vi "LoadProfiletest.vi"() -> ()   [LabVIEW 2020]
uses:
  <vilib>/Utility/file.llb/Read Delimited Spreadsheet (DBL).vi
panel:
  out "NHR error out":errorcluster
  out "VISA resource name out":refnum<visa-resource-name>
  in  "Battery Type":enum16{"30Q", "40T"}(ring)
  in  "PS VISA in":refnum<visa-resource-name>
  in  "PS type":enum16{"NHR", "ITECH"}(ring)
  in  "CyclePath":path=path "C:/Users/ga11/Desktop/VI/results/3PtestCharge.lvm" caption="Filename"
  in  "Test Time (s)":dbl format="%#.6g"
  out "Current Step":u32
  out "Time  Elapsed":dbl
  out "Time Step":dbl
  out "Load Output (A)":dbl
  out "Time Ref":dbl
  out "first row 2":dbl[](array[numeric])
  out "first row":dbl[](array[numeric])
  in  "Time file path (seconds)":path
  in  "Load file path (Amps)":path
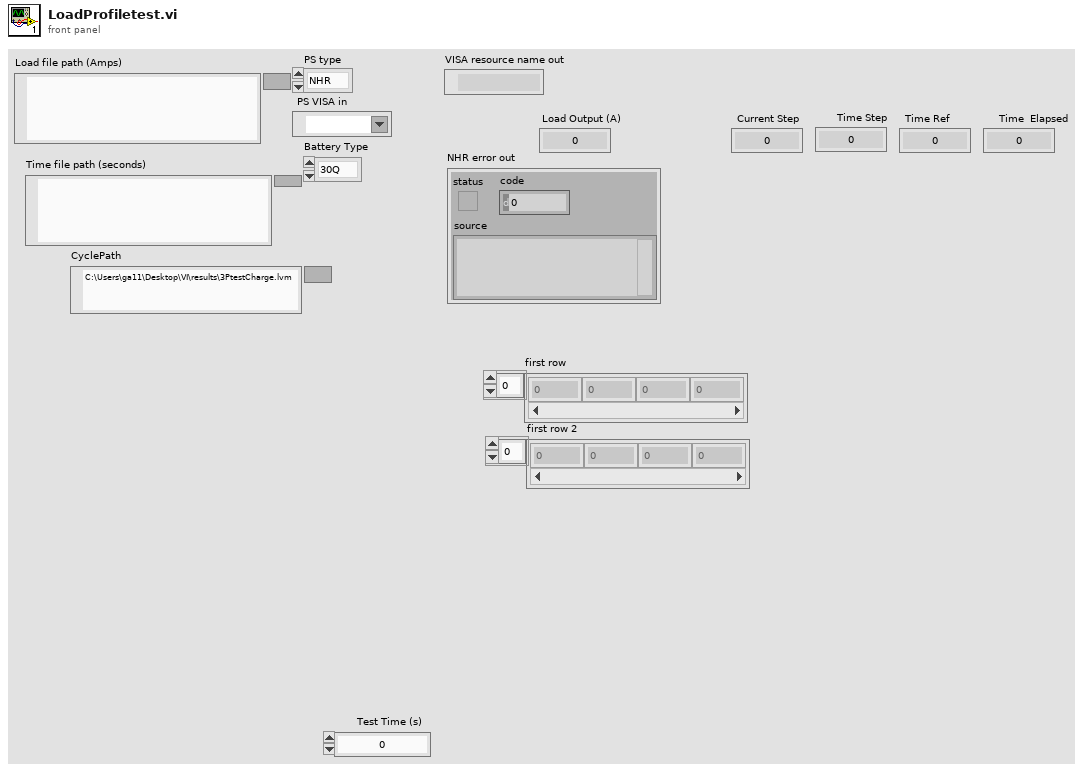
[diagram p1: front panel]
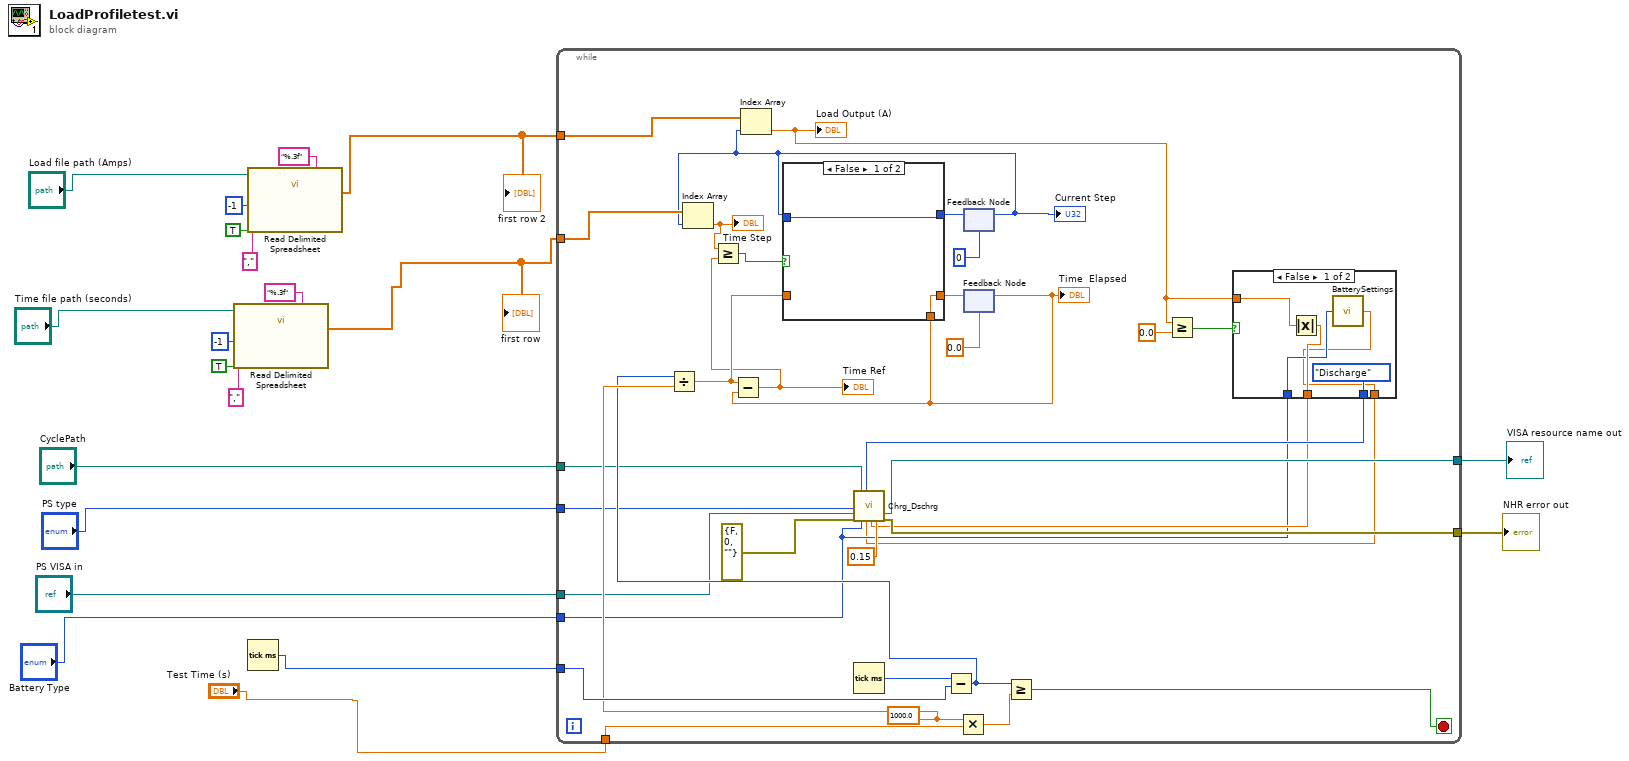
[diagram p0: block diagram]
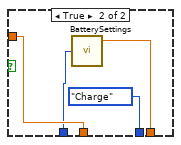
[diagram p2: hidden frame]
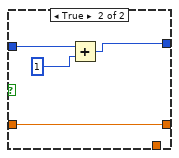
[diagram p3: hidden frame]
diagram:
  n1 = call-poly <vilib>:"Read Delimited Spreadsheet.vi"("file path (dialog if empty)"="Time file path (seconds)", "format (%.3f)"="%.3f", "number of rows (all:-1)"=-1, "transpose? (F)"=TRUE, "delimiter (\\t)"="," ("delimiter (\\t)")) -> ("first row"=w10:dbl[])  [unwired: 5 in, 5 out]
  "first row" <- w10
  n2 = call-poly <vilib>:"Read Delimited Spreadsheet.vi"("file path (dialog if empty)"="Load file path (Amps)", "format (%.3f)"="%.3f", "number of rows (all:-1)"=-1, "transpose? (F)"=TRUE, "delimiter (\\t)"="," ("delimiter (\\t)")) -> ("first row"=w9:dbl[])  [unwired: 5 in, 5 out]
  "first row 2" <- w9
  n3 = Tick Count (ms)() -> (millisecond timer value=w8:u32)
  n4 = while {
    tunnel: w10 -> [w47]
    tunnel: w9 -> [w46]
    tunnel: w8 -> [w43]
    tunnel: "Test Time (s)" -> [w41]
    tunnel: "CyclePath" -> [w33]
    tunnel: "PS type" -> [w32]
    tunnel: "PS VISA in" -> [w31]
    tunnel: "Battery Type" -> [w22]
    tunnel: [w29] -> w2
    tunnel: [w28] -> w1
    stop <- w39 stop-if-true
    w42 = 1000.0
    n5 = Tick Count (ms)() -> (millisecond timer value=w45:u32)
    n6 = Subtract(x=w45, y=w43) -> (x-y=w40:u32)
    n7 = Divide(x=w40, y=w42) -> (x/y=w53:dbl)
    n8 = Multiply(x=w42, y=w41) -> (x*y=w44:dbl)
    n9 = feedback #1(0) -> (w38:i32)
    "Current Step" <- w38
    n10 = Index Array(array=w47, index=w38) -> (element=w35:dbl)
    "Time Step" <- w35
    n11 = Index Array(array=w46, index=w38) -> (element=w24:dbl)
    "Load Output (A)" <- w24
    n12 = feedback #2(0.0) -> (w48:dbl)
    "Time  Elapsed" <- w48
    n13 = Subtract(x=w53, y=w48) -> (x-y=w37:dbl)
    "Time Ref" <- w37
    n14 = Greater Or Equal?(x=w35, y=w37) -> (x >= y?=w36:bool)
    n15 = case shown="False" w36 {
      tunnel: w53 -> [_ w68]
      tunnel: [w64 w68] -> w52
      tunnel: w48 -> [w64 _]
      tunnel: [w63 w66] -> w51
      tunnel: w38 -> [w63 w65]
      frame False {
      }
      frame True {
        n16 = Add(x=w65, y=1) -> (x+y=w66:i32)
      }
    }
    n17 = feedback-in #1(w51) -> ()
    n18 = feedback-in #2(w52) -> ()
    n19 = Greater Or Equal?(x=w40, y=w44) -> (x >= y?=w39:bool)
    n20 = Greater Or Equal?(x=w24, y=0.0) -> (x >= y?=w26:bool)
    n21 = case shown="False" w26 {
      tunnel: [enum8{"Charge", "Discharge"}."Discharge" ("Charge/discharge") enum8{"Charge", "Discharge"}."Charge" ("Charge/discharge")] -> w25
      tunnel: w24 -> [w57 w61]
      tunnel: [w56 w61] -> w23
      tunnel: w22 -> [w55 w60]
      tunnel: [w54 w59] -> w21
      frame False {
        n22 = Absolute Value(x=w57) -> (abs(x)=w56:dbl)
        n23 = call "BatterySettings.vi"("Battery Type"=w55) -> ("Min Voltage (V)"=w54:dbl)  [unwired: 2 in, 2 out]
      }
      frame True {
        n24 = call "BatterySettings.vi"("Battery Type"=w60) -> ("Max Voltage (V)"=w59:dbl)  [unwired: 2 in, 2 out]
      }
    }
    n25 = call "Chrg_Dschrg.vi"("PS type"=w32, "PS VISA in"=w31, "PS error in"=errorcluster {"status"=FALSE, "code"=0, "source"=""}, "DischargeCyclePath"=w33, "Battery Type"=w22, "Charge/discharge"=w25, "Charge/Discharge Voltage Setpoint"=w21, "Current Setpoint"=w23, "Current Cutoff"=0.15) -> ("PS VIS resource name out"=w28:refnum<visa-resource-name>, "PS error out"=w29:errorcluster)  [unwired: 7 in, 2 out]
  }
  "NHR error out" <- w2
  "VISA resource name out" <- w1
